vi "ScreenLock_SetLockState.vi"(8 "error in (no error)":errorcluster, 10 "Lock Screen":bool, 11 "OXYGEN Ref In":refnum<visa-resource-name>) -> (0 "error out":errorcluster, 1 "communication_data":T1, 3 "OXYGEN Ref Out":refnum<visa-resource-name>)   [LabVIEW 2020, in "OXYGEN_Datastream.lvlib"]
doc: "Locks/Unlocks the Screen."
uses:
  OXYGEN_Datastream.lvlib
  TypeDefs/Cluster_RawCommData.ctl
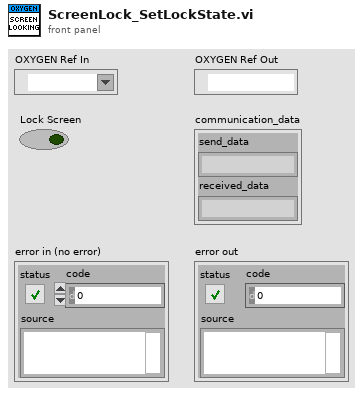
[diagram p1: front panel]
types:
  T1 = typedef "OXYGEN_Datastream.lvlib/Cluster_RawCommData.ctl" = cluster{"send_data":string, "received_data":string}
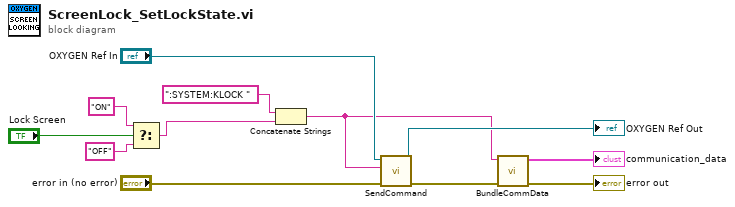
[diagram p0: block diagram]
diagram:
  n1 = Select(t="ON", s="Lock Screen", f="OFF") -> (s? t:f=w1:string)
  n2 = Concatenate Strings(":SYSTEM:KLOCK ", w1) -> (w9:string)
  n3 = call "SendCommand.vi"("error in (no error)"="error in (no error)", "String to Send"=w9, "OXY_SCPI Reseource In"="OXYGEN Ref In") -> ("error out"=w8:errorcluster, "OXY_SCPI Reseource Out"=→"OXYGEN Ref Out":refnum<visa-resource-name>)  [unwired: 7 in]
  n4 = call "BundleCommData.vi"("error in (no error)"=w8, "send_data"=w9) -> ("error out"=→"error out":errorcluster, "communication_data"=→"communication_data":T1)  [unwired: 8 in]
